vi "ShopAssortmentMain.vi"() -> ()   [LabVIEW 2020]
uses:
  #typedef_Products.ctl
  #typedef_SearchBy.ctl
  #typedef_SM_states.ctl
  #typedef_ProgramData.ctl
panel:
  in  "Sort by:":T1
  in  "Search by:":T1
  in  "Producer":string
  in  "Name":string
  in  "Product Number":dbl
  in  "Stop":bool
  out "Product":T2
  in  "Next":bool
  in  "Previous":bool
  in  "Save":bool
  in  "Remove":bool
  in  "Add":bool
  in  "Sort":bool
  in  "Search":bool
  in  "Open":bool
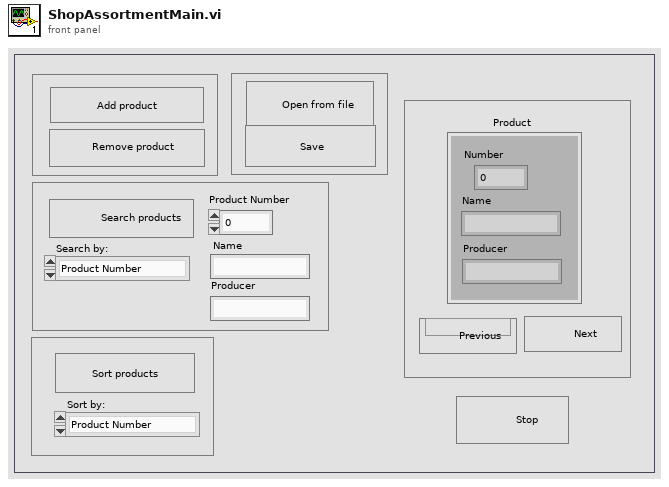
[diagram p1: front panel]
types:
  T1 = typedef "#typedef_SearchBy.ctl" = enum16{"Product Number", "Name", "Producer"}
  T2 = typedef "#typedef_Products.ctl" = cluster{"Number":dbl, "Name ":string, "Producer":string}
  T3 = typedef "#typedef_SM_states.ctl" = enum16{"Initialize", "Idle", "Add Product", "Remove Product", "Show Next", "Show Previous", "Sort products", "Search for products", "Save to file", "Open from file", "Error Handler", "Exit", "RefreshGUI"}
  T4 = typedef "#typedef_ProgramData.ctl" = cluster{"Products":T2[], "Current product":i32, "Products Data":path, "Search Product Number":dbl, "Search Name":string, "Search Producer":string}
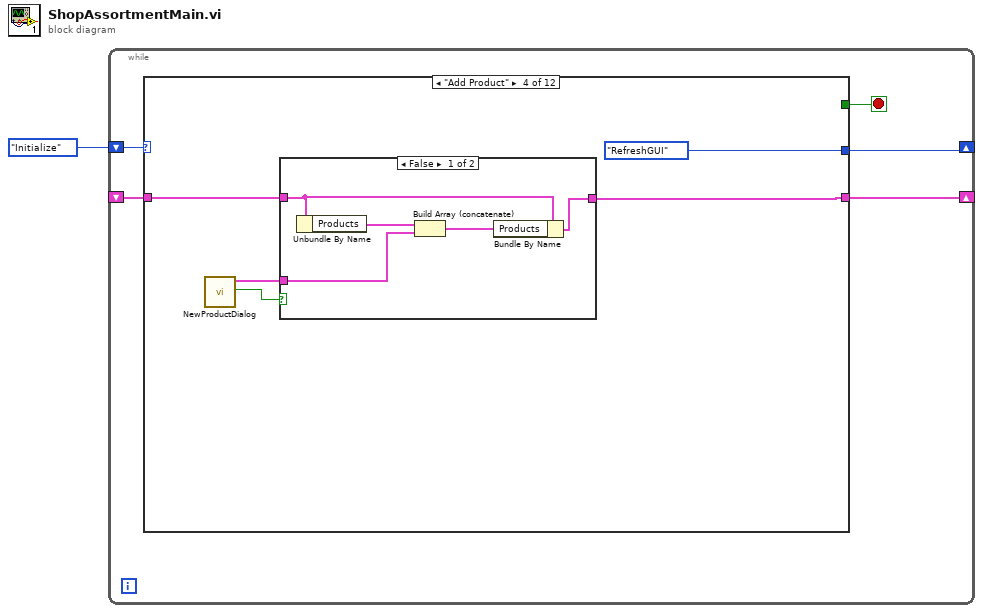
[diagram p0: block diagram]
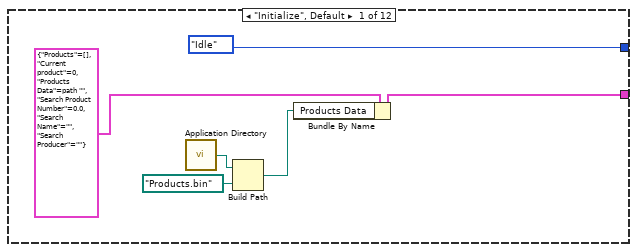
[diagram p2: hidden frame]
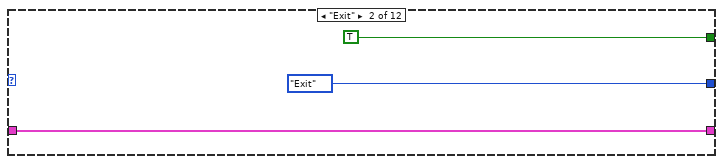
[diagram p3: hidden frame]
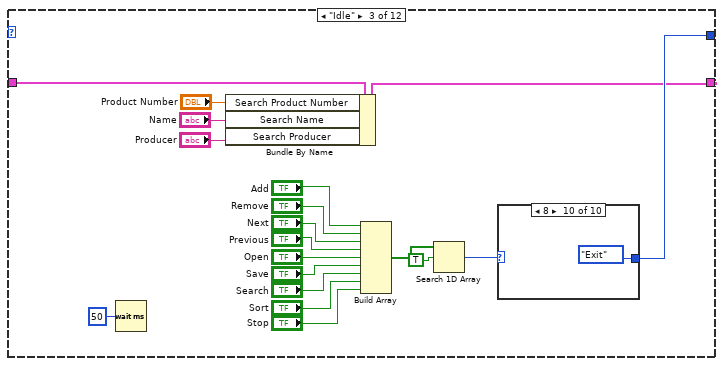
[diagram p4: hidden frame]
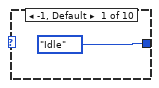
[diagram p5: hidden frame]
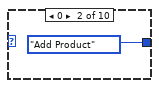
[diagram p6: hidden frame]
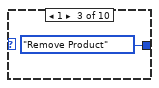
[diagram p7: hidden frame]
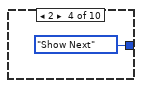
[diagram p8: hidden frame]
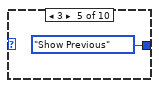
[diagram p9: hidden frame]
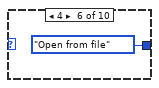
[diagram p10: hidden frame]
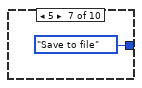
[diagram p11: hidden frame]
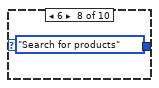
[diagram p12: hidden frame]
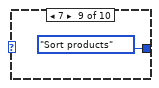
[diagram p13: hidden frame]
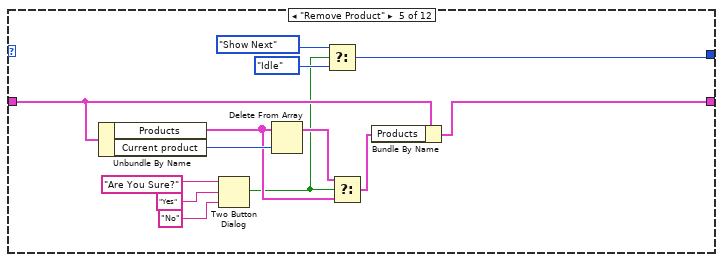
[diagram p15: hidden frame]
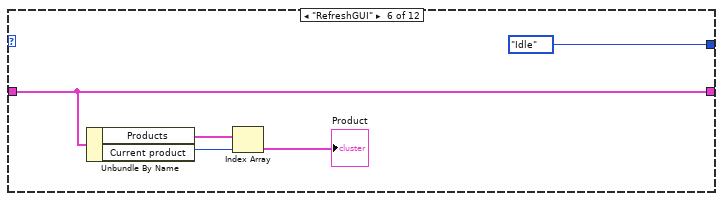
[diagram p16: hidden frame]
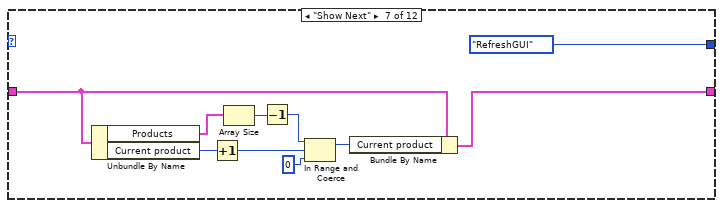
[diagram p17: hidden frame]
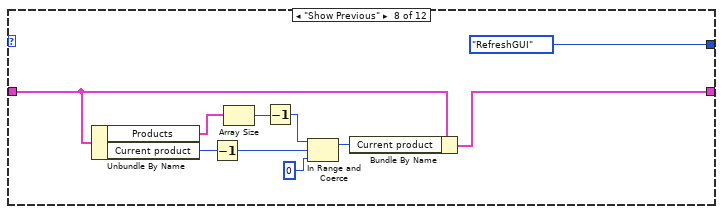
[diagram p18: hidden frame]
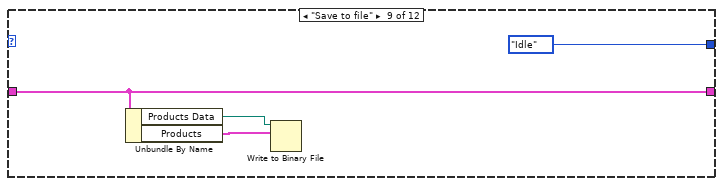
[diagram p19: hidden frame]
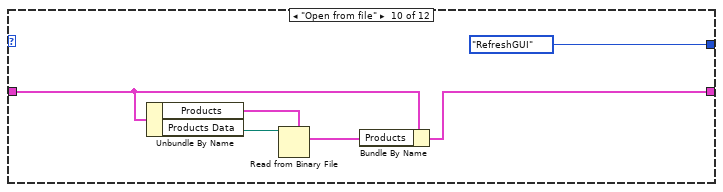
[diagram p20: hidden frame]
diagram:
  n1 = while {
    shift-right: [w4] -> _
    shift-left: #typedef_SM_states."Initialize" ("SM_States") -> [w6]
    shift-right: [w3] -> _
    shift-left: _ -> [w2]
    stop <- w5 stop-if-true
    n2 = case shown="\"Add Product\"" w6 {
      tunnel: [_ TRUE _ _ _ _ _ _ _ _ _ _] -> w5
      tunnel: [#typedef_SM_states."Idle" ("SM_States") #typedef_SM_states."Exit" ("SM_States") w23 #typedef_SM_states."RefreshGUI" ("SM_States") w58 #typedef_SM_states."Idle" ("SM_States") #typedef_SM_states."RefreshGUI" ("SM_States") #typedef_SM_states."RefreshGUI" ("SM_States") #typedef_SM_states."Idle" ("SM_States") #typedef_SM_states."RefreshGUI" ("SM_States") #typedef_SM_states."RefreshGUI" ("SM_States") #typedef_SM_states."RefreshGUI" ("SM_States")] -> w4
      tunnel: [w10 w13 w20 w47 w67 w73 w80 w90 w97 w100 w109 w151] -> w3
      tunnel: w2 -> [_ w13 w21 w48 w68 w73 w81 w91 w97 w101 w110 w152]
      frame "Initialize", Default {
        n3 = call <vilib>:"Application Directory.vi"() -> ("Application Directory"=w7:path)
        n4 = Build Path(base path=w7, name or relative path=path "Products.bin") -> (appended path=w8:path)
        n5 = Bundle By Name(cluster=T4 {"Products"=[], "Current product"=0, "Products Data"=path "", "Search Product Number"=0.0, "Search Name"="", "Search Producer"=""} ("Program data"), "Products Data"=w8) -> (w10:T4)
      }
      frame "Exit" {
      }
      frame "Idle" {
        n6 = Wait (ms)(milliseconds to wait=u32 50) -> ()  [unwired: 1 out]
        n7 = Bundle By Name(cluster=w21, "Search Product Number"="Product Number", "Search Name"="Name", "Search Producer"="Producer") -> (w20:T4)
        n8 = Build Array("Add", "Remove", "Next", "Previous", "Open", "Save", "Search", "Sort", "Stop") -> (w26:bool[])
        n9 = Search 1D Array(1D array=w26, element=TRUE) -> (index of element=w24:i32)  [unwired: 1 in]
        n10 = case shown="8" w24 {
          tunnel: [#typedef_SM_states."Idle" ("SM_States") #typedef_SM_states."Add Product" ("SM_States") #typedef_SM_states."Remove Product" ("SM_States") #typedef_SM_states."Show Next" ("SM_States") #typedef_SM_states."Show Previous" ("SM_States") #typedef_SM_states."Open from file" ("SM_States") #typedef_SM_states."Save to file" ("SM_States") #typedef_SM_states."Search for products" ("SM_States") #typedef_SM_states."Sort products" ("SM_States") #typedef_SM_states."Exit" ("SM_States")] -> w23
          frame -1, Default {
          }
          frame 0 {
          }
          frame 1 {
          }
          frame 2 {
          }
          frame 3 {
          }
          frame 4 {
          }
          frame 5 {
          }
          frame 6 {
          }
          frame 7 {
          }
          frame 8 {
          }
        }
      }
      frame "Add Product" {
        n11 = call "NewProductDialog.vi"() -> ("Cancelled ?"=w45:bool, "Product 2"=w46:T2)  [unwired: 9 in, 1 out]
        n12 = case shown="False" w45 {
          tunnel: w46 -> [w53 _]
          tunnel: w48 -> [w52 w55]
          tunnel: [w51 w55] -> w47
          frame False {
            n13 = Unbundle By Name(w52) -> ("Products"=w54:T2[])
            n14 = Build Array (concatenate)(w54, w53) -> (w50:T2[])
            n15 = Bundle By Name(cluster=w52, "Products"=w50) -> (w51:T4)
          }
          frame True {
          }
        }
      }
      frame "Remove Product" {
        n16 = Unbundle By Name(w68) -> ("Products"=w60:T2[], "Current product"=w66:i32)
        n17 = Two Button Dialog(message="Are You Sure?", 1:"No" ("F button name (\"Cancel\")"), 2:"Yes" ("button name (\"OK\")")) -> (T button?=w56:bool)
        n18 = Delete From Array(array=w60, index=w66) -> (array with subset deleted=w62:T2[])  [unwired: 1 in, 1 out]
        n19 = Select(t=#typedef_SM_states."Show Next" ("SM_States"), s=w56, f=#typedef_SM_states."Idle" ("SM_States")) -> (s? t:f=w58:T3)
        n20 = Select(t=w62, s=w56, f=w60) -> (s? t:f=w61:T2[])
        n21 = Bundle By Name(cluster=w68, "Products"=w61) -> (w67:T4)
      }
      frame "RefreshGUI" {
        n22 = Unbundle By Name(w73) -> ("Products"=w72:T2[], "Current product"=w69:i32)
        n23 = Index Array(array=w72, index=w69) -> (element=→"Product":T2)
      }
      frame "Show Next" {
        n24 = Unbundle By Name(w81) -> ("Products"=w79:T2[], "Current product"=w82:i32)
        n25 = Increment(x=w82) -> (x+1=w78:i32)
        n26 = Array Size(array=w79) -> (size(s)=w75:i32)
        n27 = Decrement(x=w75) -> (x-1=w74:i32)
        n28 = In Range and Coerce(upper limit=w74, x=w78, lower limit=0) -> (coerced(x)=w76:i32)  [unwired: 1 out]
        n29 = Bundle By Name(cluster=w81, "Current product"=w76) -> (w80:T4)
      }
      frame "Show Previous" {
        n30 = Unbundle By Name(w91) -> ("Products"=w89:T2[], "Current product"=w92:i32)
        n31 = Decrement(x=w92) -> (x-1=w88:i32)
        n32 = Array Size(array=w89) -> (size(s)=w86:i32)
        n33 = Decrement(x=w86) -> (x-1=w85:i32)
        n34 = In Range and Coerce(upper limit=w85, x=w88, lower limit=0) -> (coerced(x)=w87:i32)  [unwired: 1 out]
        n35 = Bundle By Name(cluster=w91, "Current product"=w87) -> (w90:T4)
      }
      frame "Save to file" {
        n36 = Unbundle By Name(w97) -> ("Products Data"=w95:path, "Products"=w96:T2[])
        n37 = Write to Binary File(file (use dialog)=w95, data=w96) -> ()  [unwired: 4 in, 3 out]
      }
      frame "Open from file" {
        n38 = Unbundle By Name(w101) -> ("Products"=w99:T2[], "Products Data"=w103:path)
        n39 = Read from Binary File(5:w99, 11:w103) -> (2:w102:T2[])  [unwired: 4 in, 3 out]
        n40 = Bundle By Name(cluster=w101, "Products"=w102) -> (w100:T4)
      }
      frame "Search for products" {
        n41 = Unbundle By Name(w110) -> ("Products"=w112:T2[], "Search Product Number"=w105:dbl, "Search Name"=w106:string, "Search Producer"=w104:string)
        n42 = Array Size(array=w112) -> (size(s)=w111:i32)
        n43 = case shown="\"Producer\"" "Search by:" {
          tunnel: w105 -> [w117 _ _]
          tunnel: w112 -> [w116 w129 w141]
          tunnel: w111 -> [w115 w128 w140]
          tunnel: [w114 w127 w139] -> w108
          tunnel: w106 -> [_ w126 _]
          tunnel: w104 -> [_ _ w138]
          frame "Product Number" {
            n44 = while {
              tunnel: w116 -> [w125] mode=indexing
              tunnel: w117 -> [w123]
              tunnel: w115 -> [w120]
              tunnel: [w119] -> w114
              i -> [w119]
              stop <- w121 stop-if-true
              n45 = Unbundle By Name(w125) -> ("Number"=w124:dbl)
              n46 = Equal?(x=w120, y=w119) -> (x = y?=w118:bool)
              n47 = Equal?(x=w124, y=w123) -> (x = y?=w122:bool)
              n48 = Or(x=w122, y=w118) -> (x .or. y?=w121:bool)
            }
          }
          frame "Name" {
            n49 = while {
              tunnel: w129 -> [w137] mode=indexing
              tunnel: w128 -> [w133]
              tunnel: [w132] -> w127
              tunnel: w126 -> [w130]
              i -> [w132]
              stop <- w134 stop-if-true
              n50 = Unbundle By Name(w137) -> ("Name"=w136:string)
              n51 = Equal?(x=w133, y=w132) -> (x = y?=w131:bool)
              n52 = Equal?(x=w136, y=w130) -> (x = y?=w135:bool)
              n53 = Or(x=w135, y=w131) -> (x .or. y?=w134:bool)
            }
          }
          frame "Producer" {
            n54 = while {
              tunnel: w141 -> [w149] mode=indexing
              tunnel: w140 -> [w145]
              tunnel: [w144] -> w139
              tunnel: w138 -> [w142]
              i -> [w144]
              stop <- w146 stop-if-true
              n55 = Unbundle By Name(w149) -> ("Producer"=w148:string)
              n56 = Equal?(x=w145, y=w144) -> (x = y?=w143:bool)
              n57 = Equal?(x=w148, y=w142) -> (x = y?=w147:bool)
              n58 = Or(x=w147, y=w143) -> (x .or. y?=w146:bool)
            }
          }
        }
        n59 = Bundle By Name(cluster=w110, "Current product"=w108) -> (w109:T4)
      }
      frame "Sort products" {
        n60 = Unbundle By Name(w152) -> ("Products"=w155:T2[])
        n61 = case shown="\"Product Number\"" "Sort by:" {
          tunnel: w155 -> [w159 w168 w177]
          tunnel: [w156 w165 w174] -> w153
          frame "Product Number" {
            n62 = for {
              tunnel: w159 -> [w162] mode=indexing
              tunnel: [w163] -> w158 mode=indexing
              n63 = Unbundle By Name(w162) -> ("Number"=w164:dbl)
              n64 = Bundle("Number"=w164, "Product"=w162) -> (w163:cluster{"Number":dbl, "Product":T2})  [unwired: 1 in]
            }
            n65 = Sort 1D Array(array=w158) -> (sorted array=w157:cluster{"Number":dbl, "Product":T2}[])
            n66 = for {
              tunnel: w157 -> [w161] mode=indexing
              tunnel: [w160] -> w156 mode=indexing
              n67 = Unbundle(w161) -> ("Product"=w160:T2)  [unwired: 1 out]
            }
          }
          frame "Name" {
            n68 = for {
              tunnel: w168 -> [w171] mode=indexing
              tunnel: [w172] -> w167 mode=indexing
              n69 = Unbundle By Name(w171) -> ("Name"=w173:string)
              n70 = Bundle("Name"=w173, "Product"=w171) -> (w172:cluster{"Name ":string, "Product":T2})  [unwired: 1 in]
            }
            n71 = Sort 1D Array(array=w167) -> (sorted array=w166:cluster{"Name ":string, "Product":T2}[])
            n72 = for {
              tunnel: w166 -> [w170] mode=indexing
              tunnel: [w169] -> w165 mode=indexing
              n73 = Unbundle(w170) -> ("Product"=w169:T2)  [unwired: 1 out]
            }
          }
          frame "Producer" {
            n74 = for {
              tunnel: w177 -> [w180] mode=indexing
              tunnel: [w181] -> w176 mode=indexing
              n75 = Unbundle By Name(w180) -> ("Producer"=w182:string)
              n76 = Bundle("Producer"=w182, "Product"=w180) -> (w181:cluster{"Producer":string, "Product":T2})  [unwired: 1 in]
            }
            n77 = Sort 1D Array(array=w176) -> (sorted array=w175:cluster{"Producer":string, "Product":T2}[])
            n78 = for {
              tunnel: w175 -> [w179] mode=indexing
              tunnel: [w178] -> w174 mode=indexing
              n79 = Unbundle(w179) -> ("Product"=w178:T2)  [unwired: 1 out]
            }
          }
        }
        n80 = Bundle By Name(cluster=w152, "Products"=w153) -> (w151:T4)
      }
    }
  }
